vi "http.get.vi"(6 "specific headers in":cluster{"header":string, "value":string}[](array[cluster]), 8 "error in":errorcluster, 10 "Path":string, 11 "Nominal Client in":refnum<class "Nominal Client.lvclass">) -> (0 "error out":errorcluster, 2 "Response":string, 3 "Nominal Client out":refnum<class "Nominal Client.lvclass">)   [LabVIEW 2020, in "Nominal Client.lvclass"]
uses:
  Nominal Client.lvclass
  Nominal Client.lvclass/Nominal Client.ctl
  <vilib>/JDP Science/JSONtext/LVClass Serializer/JSONtext LVClass Serializer.lvclass
  submodules/reqwest-labview/lv-src/reqwest/reqwest.lvclass
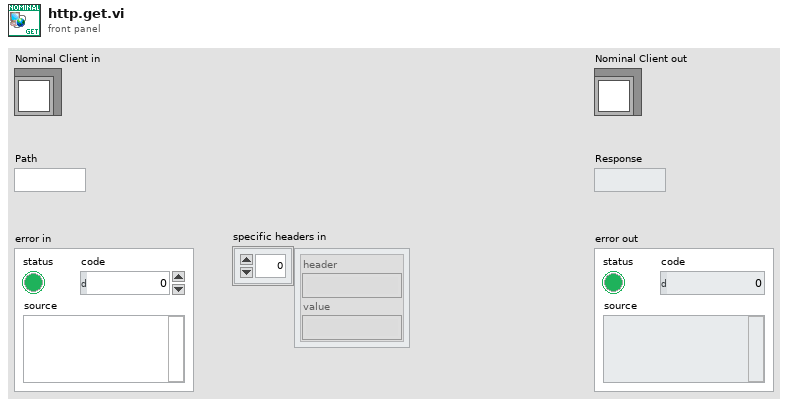
[diagram p1: front panel]
types:
  T1 = typedef "Nominal Client.lvclass/private_data.ctl" = cluster{"API Token":string, "workspace":refnum<class "workspace.lvclass">, "Available Workspaces":refnum<class "workspace.lvclass">[], "reqwest":refnum<class "reqwest.lvclass">, "timeout ms":i32}
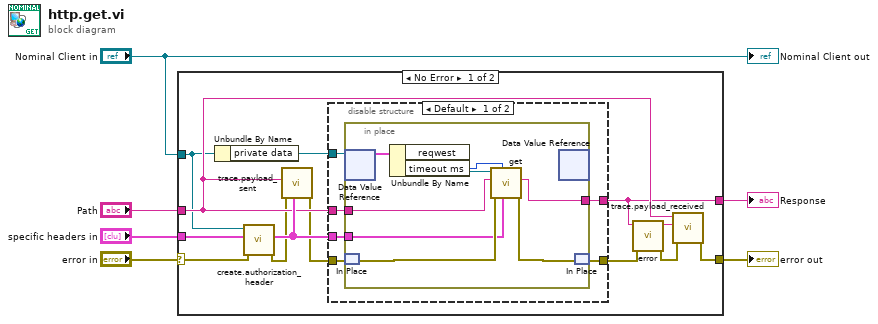
[diagram p0: block diagram]
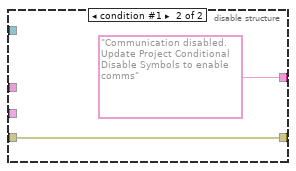
[diagram p2: hidden frame]
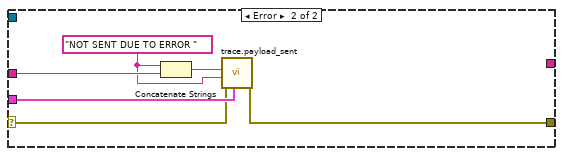
[diagram p3: hidden frame]
diagram:
  n1 = case shown="No Error" "error in" {
    selector: "error in" -> [w15 w40]
    tunnel: "Nominal Client in" -> [w11 _]
    tunnel: "specific headers in" -> [w17 w41]
    tunnel: "Path" -> [w16 w38]
    tunnel: [w13 _] -> w2
    tunnel: [w7 w39] -> w1
    frame No Error {
      n2 = Unbundle By Name(w11) -> ("private data"=w18:refnum<data-value>)
      n3 = call "create.authorization_header.vi"("error in"=w15, "specific headers in"=w17, "Nominal Client in"=w11) -> ("error out"=w10:errorcluster, "specific headers out"=w19:cluster{"header":string, "value":string}[])  [unwired: 6 in, 1 out]
      n4 = call "trace.payload_sent.vi"("Headers"=w19, "dataflow error in"=w10, "Path"=w16) -> ("dataflow error out"=w9:errorcluster)  [unwired: 8 in]
      n5 = disable-structure shown="Default" {
        disable-tunnel: w19 -> [w25 _]
        disable-tunnel: w18 -> [w24 _]
        disable-tunnel: w16 -> [w23 _]
        disable-tunnel: w9 -> [w22 w34]
        disable-tunnel: [w21 "Communication disabled. Update Project Conditional Disable Symbols to enable comms" ("REST Response")] -> w13
        disable-tunnel: [w20 w34] -> w12
        frame condition #0 (active) {
          n6 = in-place {
            in-place-border: w25 -> [w30]
            in-place-border: [w31] -> w21
            in-place-border: w23 -> [w29]
            n7 = in-place-dvr #1(w24) -> (w33:T1)  [unwired: 1 out]
            n8 = in-place-match #2(w22) -> (w32:errorcluster)
            n9 = Unbundle By Name(w33) -> ("reqwest"=w27:refnum<class "reqwest.lvclass">, "timeout ms"=w26:i32)
            n10 = call "get.vi"("request specific headers"=w30, "timeout (ms)"=w26, "error in (no error)"=w32, "path"=w29, "reqwest in"=w27) -> ("error out"=w28:errorcluster, "response"=w31:string)  [unwired: 4 in, 1 out]
            n11 = in-place-dvr #1() -> ()  [unwired: 1 in, 2 out]
            n12 = in-place-match #2(w28) -> (w20:errorcluster)
          }
        }
        frame condition #1 {
        }
      }
      n13 = call "error.vi"("error in"=w12, "REST Response"=w13) -> ("error out"=w8:errorcluster, "Error Formatted Response"=w14:string)  [unwired: 8 in]
      n14 = call "trace.payload_received.vi"("dataflow error in"=w8, "Response"=w14, "Path"=w16) -> ("dataflow error out"=w7:errorcluster)  [unwired: 8 in]
    }
    frame Error {
      w36 = "NOT SENT DUE TO ERROR " ("string")
      n15 = Concatenate Strings(w36, w38) -> (w37:string)
      n16 = call "trace.payload_sent.vi"("Headers"=w41, "dataflow error in"=w40, "Request Body"=w36, "Path"=w37) -> ("dataflow error out"=w39:errorcluster)  [unwired: 7 in]
    }
  }
  "error out" <- w1
  "Response" <- w2
  "Nominal Client out" <- "Nominal Client in"
